vi "Teardown.vi"(8 "error in (no error)":errorcluster, 11 "Configuration File Interface Test In":refnum<class "Configuration File Base Interface Test.lvclass">) -> (0 "error out":errorcluster, 3 "Configuration File Interface Test Out":refnum<class "Configuration File Base Interface Test.lvclass">)   [LabVIEW 2020, in "Configuration File Base Interface Test.lvclass"]
uses:
  Configuration File Base Interface Test.lvclass
  C:/Git/astemes-triarc-framework/tests/Configuration Interface Test/Configuration Interface Test.lvclass
  Mock Configurable Base/Mock Configurable Base.lvclass
  C:/Git/astemes-triarc-framework/source/Framework/Base/Base.lvclass
  source/Framework/Base/Base.lvclass/Base.ctl
  Configuration File Base Interface Test.lvclass/Configuration File Base Interface Test.ctl
  Configuration Interface Test/Configuration Interface Test.lvclass
  source/Framework/Base/Base.lvclass
  C:/Program Files (x86)/National Instruments/LabVIEW 2020/vi.lib/Astemes/LUnit/Test Case.lvclass
  C:/Git/astemes-triarc-framework/tests/Configuration File Interface Test/Configuration File Base Interface Test.lvclass
  C:/Git/astemes-triarc-framework/source/Framework/Configuration File/Configuration File.lvclass
  C:/Git/astemes-triarc-framework/source/Framework/Configuration/Configuration.lvclass
  C:/Git/astemes-triarc-framework/tests/Mock Configurable Base/Mock Configurable Base.lvclass
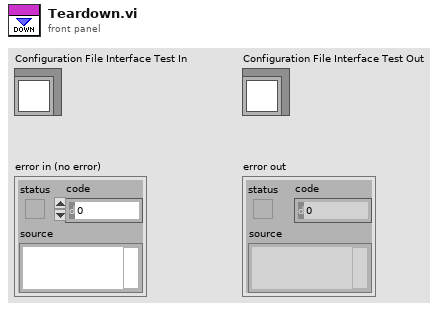
[diagram p1: front panel]
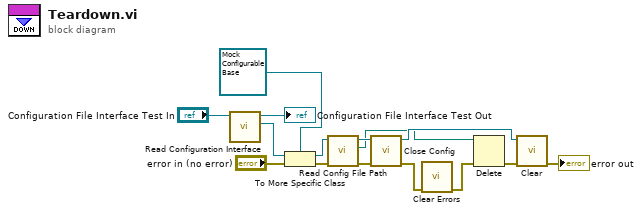
[diagram p0: block diagram]
diagram:
  n1 = call "Read Configuration Interface.vi"("Configuration Interface Test In"="Configuration File Interface Test In") -> ("Configuration"=w13:refnum<class "Configuration.lvclass">, "Configuration Interface Test Out"=→"Configuration File Interface Test Out":refnum<class "Configuration File Base Interface Test.lvclass">)  [unwired: 9 in]
  n2 = To More Specific Class(target class=refnum<class "Mock Configurable Base.lvclass"> refnum ("Mock Configurable.lvclass"), reference=w13, error in="error in (no error)") -> (specific class reference=w2:refnum<class "Mock Configurable Base.lvclass">, error out=w4:errorcluster)
  n3 = call "Read Config File Path.vi"("error in (no error)"=w4, "Base In"=w2) -> ("error out"=w7:errorcluster, "Config File Path"=w5:path, "Base Out"=w6:refnum<class "Mock Configurable Base.lvclass">)  [unwired: 7 in]
  n4 = call-dynamic "Close Config.vi"("error in (no error)"=w7, "Configuration File File In"=w6) -> ("error out"=w10:errorcluster, "Configuration File File Out"=w9:refnum<class "Mock Configurable Base.lvclass">)  [unwired: 8 in]
  n5 = call <vilib>:"Clear Errors.vi"("error in (no error)"=w10) -> ("error out"=w1:errorcluster)  [unwired: 5 in, 1 out]
  n6 = Delete(path (use dialog)=w5, error in=w1) -> (error out=w11:errorcluster)  [unwired: 3 in, 2 out]
  n7 = call-dynamic "Clear.vi"("error in (no error)"=w11, "Base In"=w9) -> ("error out"=→"error out":errorcluster)  [unwired: 9 in]
